vi "ATM Main.vi"() -> ()   [LabVIEW 2019]
doc: "Use this template to build a simple state machine design pattern. Each state executes code and determines which state to transition to."
uses:
  controls/ATM State.ctl
panel:
  in  "Shut Down":bool
  in  "Amount":dbl
  in  "Name":string
  in  "Enter":bool
  in  "Pin":string
  in  "Card":bool
  out "Atm Display":string caption="Display"
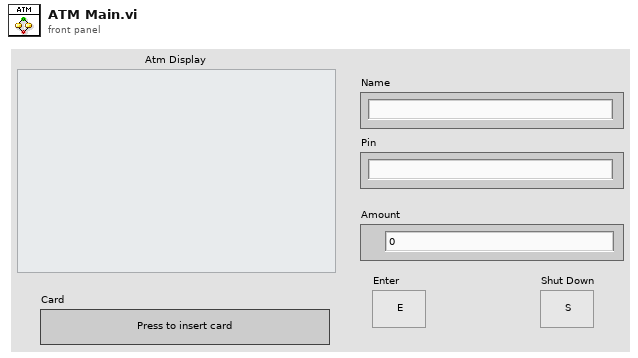
[diagram p1: front panel]
types:
  T1 = typedef "ATM State.ctl" = enum16{"Initialize", "Wait for Event", "Credentials", "Check Credentials", "Withdraw", "Withdraw Message", "Incorrect Pin", "Exit"}
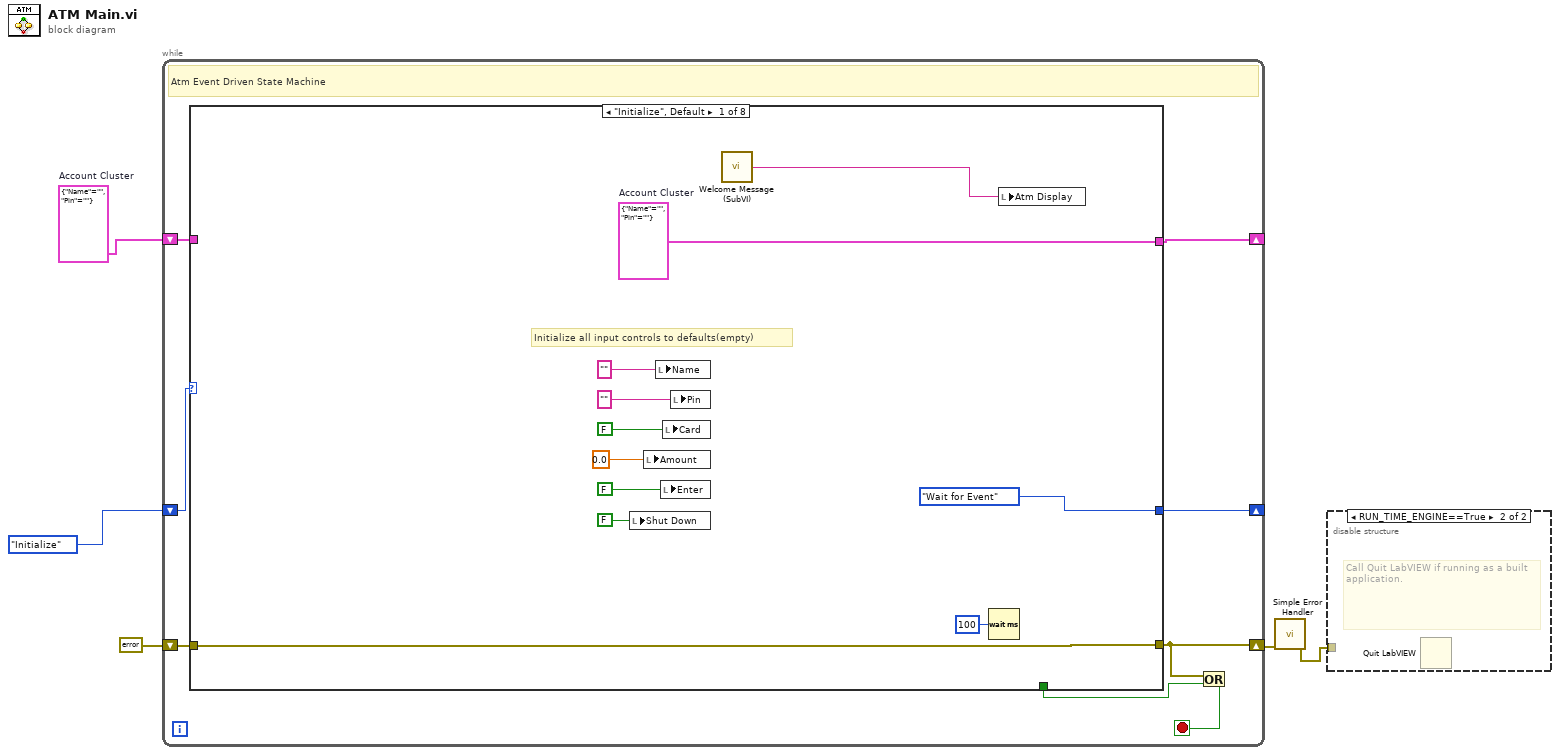
[diagram p0: block diagram]
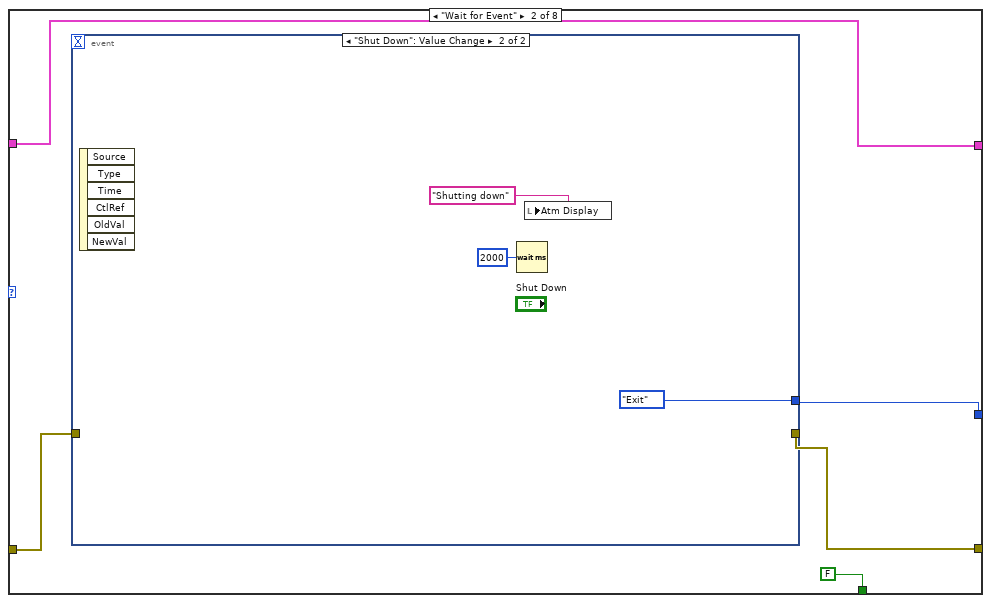
[diagram p3: hidden frame]
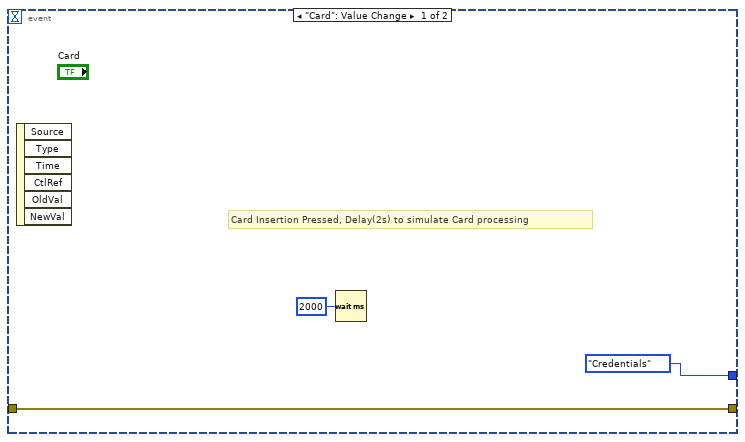
[diagram p4: hidden frame]
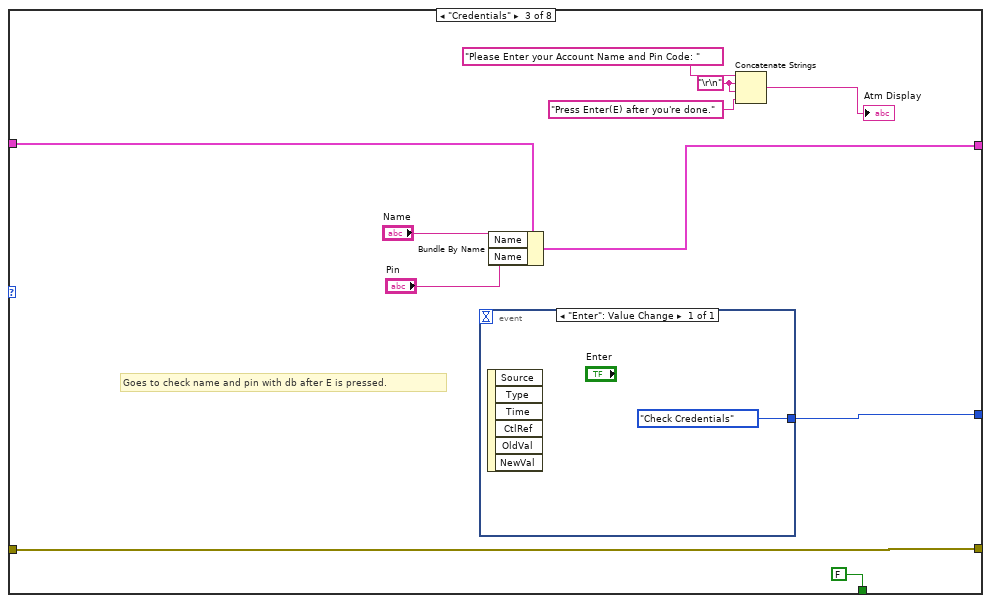
[diagram p5: hidden frame]
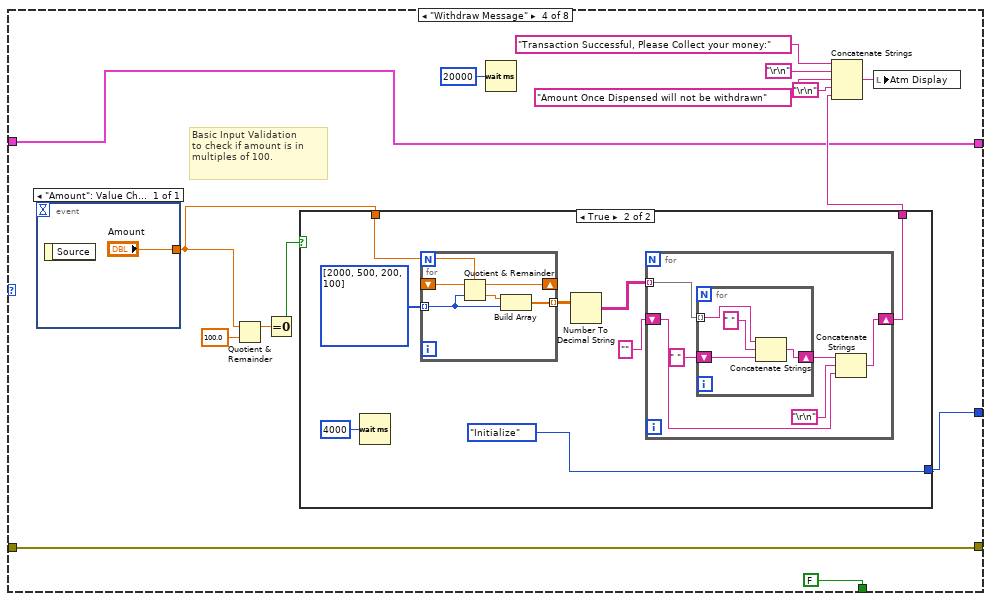
[diagram p6: hidden frame]
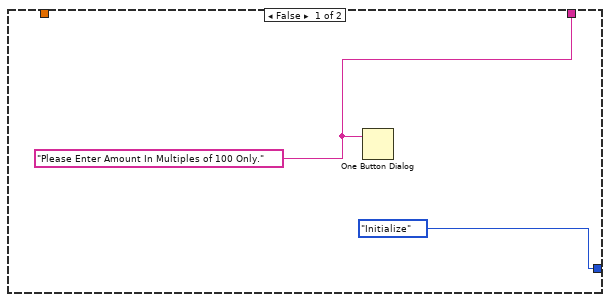
[diagram p7: hidden frame]
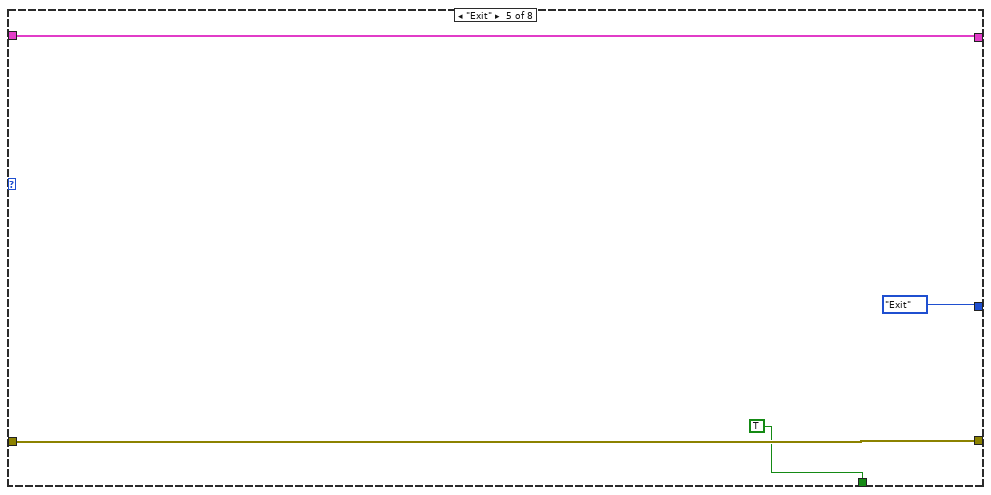
[diagram p8: hidden frame]
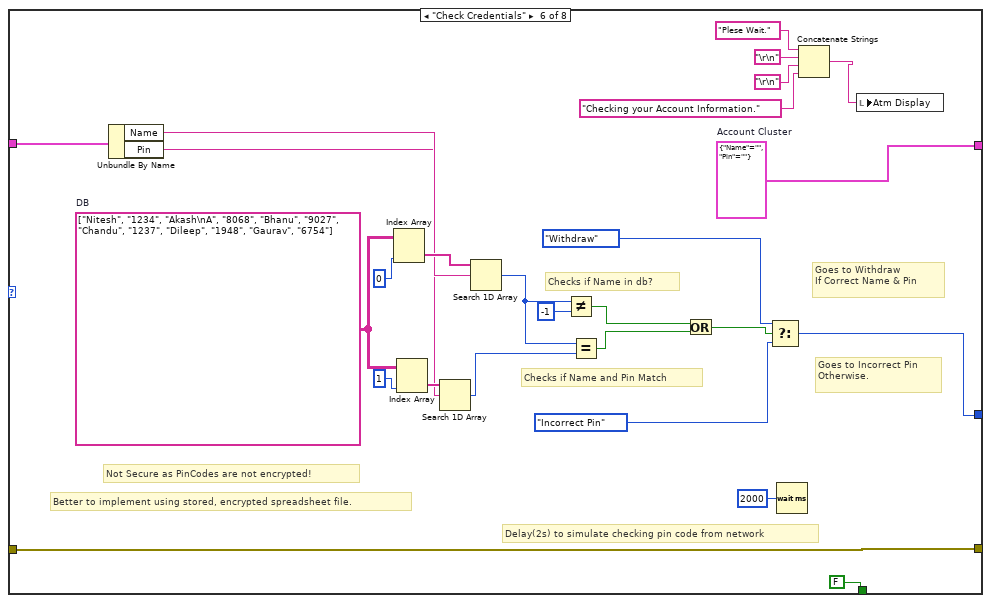
[diagram p9: hidden frame]
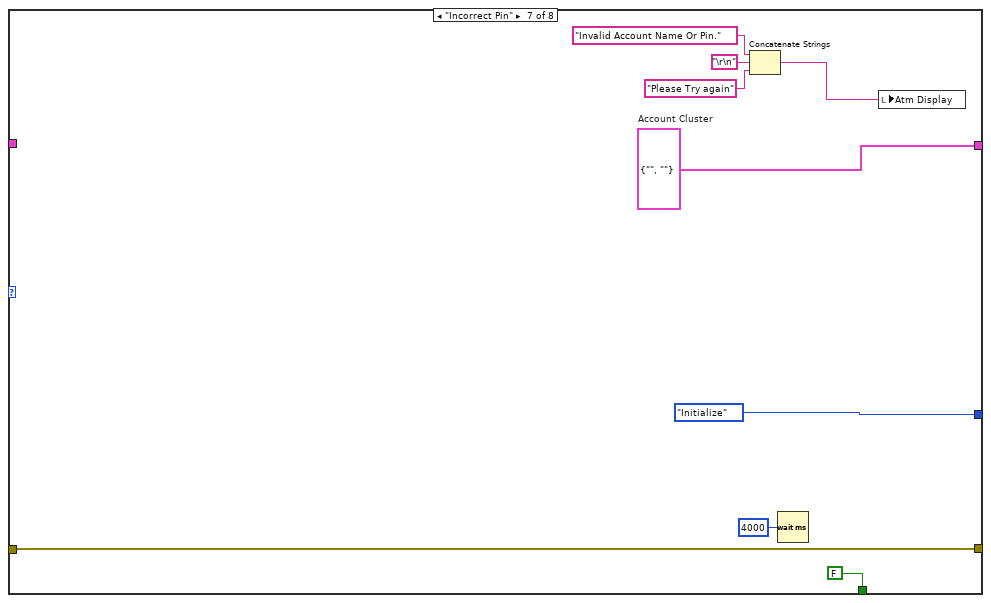
[diagram p10: hidden frame]
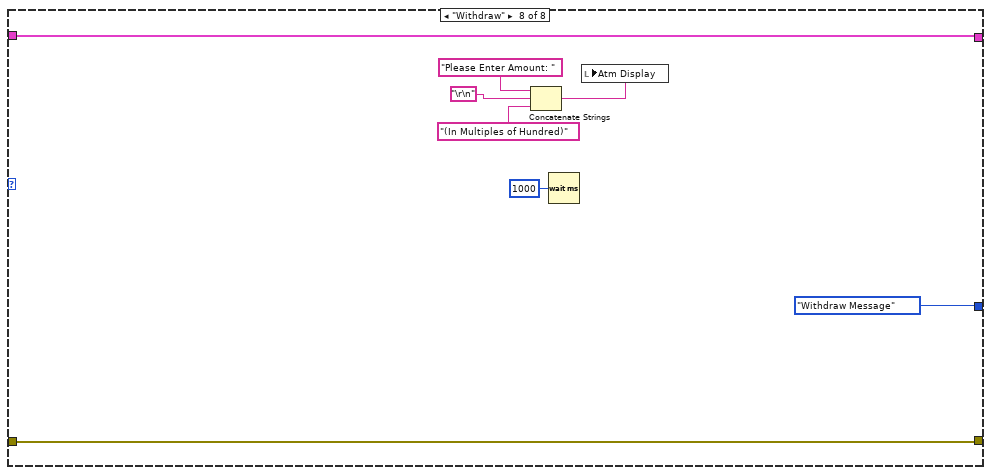
[diagram p11: hidden frame]
diagram:
  w1 = cluster{"Name":string, "Pin":string} {"Name"="", "Pin"=""}  # Account Cluster
  n1 = while {
    shift-right: [w8] -> w4
    shift-left: errorcluster {"status"=FALSE, "code"=0, "source"=""} ("error constant") -> [w13]
    shift-right: [w11] -> _
    shift-left: ATM_State."Initialize" ("States") -> [w12]
    shift-right: [w10] -> _
    shift-left: w1 -> [w9]
    stop <- w6 stop-if-true
    # "Atm Event Driven State Machine"
    n2 = case shown="\"Initialize\", Default" w12 {
      tunnel: w13 -> [w21 w29 w39 w53 w92 w102 w121 w128]
      tunnel: [w21 w28 w39 w53 w92 w102 w121 w128] -> w8
      tunnel: [ATM_State."Wait for Event" ("States") w27 w40 w52 ATM_State."Exit" ("States") w105 ATM_State."Initialize" ("States") ATM_State."Withdraw Message" ("States")] -> w11
      tunnel: [w22 w26 w42 w54 w91 w101 w127 w129] -> w10
      tunnel: w9 -> [_ w26 w41 w54 w91 w108 _ w129]
      tunnel: [_ FALSE FALSE FALSE TRUE FALSE FALSE _] -> w7
      frame "Initialize", Default {
        w22 = cluster{"Name":string, "Pin":string} {"Name"="", "Pin"=""}  # Account Cluster
        # "Initialize all input controls to defaults(empty)"
        n3 = local write "Shut Down"(FALSE ("Shut Down")) -> ()
        n4 = local write "Amount"(0.0 ("Amount")) -> ()
        n5 = local write "Name"("" ("Name")) -> ()
        n6 = local write "Enter"(FALSE) -> ()
        n7 = local write "Card"(FALSE) -> ()
        n8 = local write "Pin"("" ("Pin")) -> ()
        n9 = call "Welcome Message (SubVI).vi"() -> ("String"=w19:string)
        n10 = Wait (ms)(milliseconds to wait=u32 100) -> ()  [unwired: 1 out]
        n11 = local write "Atm Display"(w19) -> ()
      }
      frame "Wait for Event" {
        n12 = event shown="[1] \"Shut Down\": Value Change" {
          selector: _ -> [_ _]
          dyn-events: _ -> [_ _]
          timeout: _ -> [_ _]
          tunnel: w29 -> [w30 _]
          tunnel: [w30 _] -> w28
          tunnel: [ATM_State."Credentials" ("States") ATM_State."Exit" ("States")] -> w27
          event "Card": Value Change {
            # "Card Insertion Pressed, Delay(2s) to simulate Card processing"
            n13 = event-data() -> ()  [unwired: 1 in, 6 out]
            n14 = Wait (ms)(milliseconds to wait=u32 2000) -> ()  [unwired: 1 out]
          }
          event "Shut Down": Value Change {
            n15 = event-data() -> ()  [unwired: 1 in, 6 out]
            n16 = Wait (ms)(milliseconds to wait=u32 2000) -> ()  [unwired: 1 out]
            n17 = local write "Atm Display"("Shutting down" ("Atm Display")) -> ()
          }
        }
      }
      frame "Credentials" {
        w36 = "\r\n"
        # "Goes to check name and pin with db after E is pressed."
        n18 = event shown="[0] \"Enter\": Value Change" {
          selector: _ -> [_]
          dyn-events: _ -> [_]
          timeout: _ -> [_]
          tunnel: [ATM_State."Check Credentials" ("States")] -> w40
          event "Enter": Value Change {
            n19 = event-data() -> ()  [unwired: 1 in, 6 out]
          }
        }
        n20 = Bundle By Name(cluster=w41, "Name"="Name", "Name"="Pin") -> (w42:cluster{"Name":string, "Pin":string})
        n21 = Concatenate Strings("Please Enter your Account Name and Pin Code: ", w36, w36, "Press Enter(E) after you're done." ("string")) -> (→"Atm Display":string)
      }
      frame "Withdraw Message" {
        # "Basic Input Validation\nto check if amount is in\nmultiples of 100."
        n22 = event shown="[0] \"Amount\": Value Change" {
          selector: _ -> [_]
          dyn-events: _ -> [_]
          timeout: _ -> [_]
          tunnel: ["Amount"] -> w49
          event "Amount": Value Change {
            n23 = event-data() -> ()  [unwired: 1 in, 1 out]
          }
        }
        n24 = Quotient & Remainder(x=w49, y=100.0) -> (x-y*floor(x/y)=w61:dbl)  [unwired: 1 out]
        n25 = Equal To 0?(x=w61) -> (x = 0?=w60:bool)
        n26 = case shown="True" w60 {
          tunnel: w49 -> [_ w69]
          tunnel: [w64 w68] -> w59
          tunnel: [ATM_State."Initialize" ("States") ATM_State."Initialize" ("States")] -> w52
          frame False {
            w64 = "Please Enter Amount In Multiples of 100 Only."
            n27 = One Button Dialog(message=w64) -> ()  [unwired: 1 in, 1 out]
          }
          frame True {
            n28 = Wait (ms)(milliseconds to wait=u32 4000) -> ()  [unwired: 1 out]
            n29 = for {
              tunnel: i32[] [2000, 500, 200, 100] -> [w87] mode=indexing
              shift-right: [w85] -> _
              shift-left: w69 -> [w88]
              tunnel: [w86] -> w72 mode=indexing
              n30 = Quotient & Remainder(x=w88, y=w87) -> (x-y*floor(x/y)=w85:dbl, floor(x/y)=w84:dbl)
              n31 = Build Array(w84, w87) -> (w86:dbl[])
            }
            n32 = Number To Decimal String(number=w72) -> (decimal integer string=w70:string[][])  [unwired: 1 in]
            n33 = for {
              shift-right: [w74] -> w68
              shift-left: "" -> [w79]
              tunnel: w70 -> [w77] mode=indexing
              n34 = for {
                tunnel: w77 -> [w83] mode=indexing
                shift-right: [w80] -> w75
                shift-left: " " -> [w81]
                n35 = Concatenate Strings(w83, " ", w81) -> (w80:string)
              }
              n36 = Concatenate Strings(w75, "\r\n", w79) -> (w74:string)
            }
          }
        }
        n37 = Wait (ms)(milliseconds to wait=u32 20000) -> ()  [unwired: 1 out]
        n38 = Concatenate Strings("Transaction Successful, Please Collect your money:" ("string"), "\r\n", "Amount Once Dispensed will not be withdrawn" ("string"), "\r\n", w59) -> (w50:string)
        n39 = local write "Atm Display"(w50) -> ()
      }
      frame "Exit" {
      }
      frame "Check Credentials" {
        w101 = cluster{"Name":string, "Pin":string} {"Name"="", "Pin"=""}  # Account Cluster
        w113 = string[][] [["Nitesh", "1234"], ["Akash\nA", "8068"], ["Bhanu", "9027"], ["Chandu", "1237"], ["Dileep", "1948"], ["Gaurav", "6754"]]  # DB
        # "Checks if Name and Pin Match"
        # "Checks if Name in db?"
        # "Goes to Incorrect Pin\nOtherwise."
        # "Goes to Withdraw\nIf Correct Name & Pin"
        # "Not Secure as PinCodes are not encrypted!"
        # "Better to implement using stored, encrypted spreadsheet file."
        # "Delay(2s) to simulate checking pin code from network"
        n40 = Unbundle By Name(w108) -> ("Name"=w107:string, "Pin"=w106:string)
        n41 = Index Array(array=w113, index (col)=0 ("disabled index (col)")) -> (element=w112:string[])  [unwired: 1 in]
        n42 = Index Array(array=w113, index (col)=1 ("disabled index (col)")) -> (element=w109:string[])  [unwired: 1 in]
        n43 = Search 1D Array(1D array=w109, element=w106) -> (index of element=w96:i32)  [unwired: 1 in]
        n44 = Search 1D Array(1D array=w112, element=w107) -> (index of element=w97:i32)  [unwired: 1 in]
        n45 = Not Equal?(x=w97, y=-1) -> (x != y?=w94:bool)
        n46 = Equal?(x=w97, y=w96) -> (x = y?=w95:bool)
        n47 = Or(x=w94, y=w95) -> (x .or. y?=w93:bool)
        n48 = Select(t=ATM_State."Withdraw" ("States"), s=w93, f=ATM_State."Incorrect Pin" ("States")) -> (s? t:f=w105:T1)
        n49 = Wait (ms)(milliseconds to wait=u32 2000) -> ()  [unwired: 1 out]
        n50 = Concatenate Strings("Plese Wait.", "\r\n", "\r\n", "Checking your Account Information.") -> (w99:string)
        n51 = local write "Atm Display"(w99) -> ()
      }
      frame "Incorrect Pin" {
        w127 = cluster{"Name":string, "Pin":string} {"Name"="", "Pin"=""}  # Account Cluster
        n52 = Concatenate Strings("Invalid Account Name Or Pin.", "\r\n", "Please Try again") -> (w119:string)
        n53 = Wait (ms)(milliseconds to wait=u32 4000) -> ()  [unwired: 1 out]
        n54 = local write "Atm Display"(w119) -> ()
      }
      frame "Withdraw" {
        n55 = Concatenate Strings("Please Enter Amount: ", "\r\n", "(In Multiples of Hundred)") -> (w135:string)
        n56 = Wait (ms)(milliseconds to wait=u32 1000) -> ()  [unwired: 1 out]
        n57 = local write "Atm Display"(w135) -> ()
      }
    }
    n58 = Or(x=w8, y=w7) -> (x .or. y?=w6:bool)
  }
  n59 = call <vilib>:"Simple Error Handler.vi"("error in (no error)"=w4) -> ("error out"=w3:errorcluster)  [unwired: 4 in, 4 out]
  n60 = disable-structure shown="RUN_TIME_ENGINE==True" {
    disable-tunnel: w3 -> [_ _]
    frame condition #0 (active) {
    }
    frame condition #1 {
      # "Call Quit LabVIEW if running as a built application."
      n61 = Quit LabVIEW() -> ()  [unwired: 1 in]
    }
  }
